vi "GetText.vi"(8 "error in":errorcluster, 11 "Thermo Channel in":refnum<class "Thermo Channel.lvclass">) -> (0 "error out":errorcluster, 1 "additional text":string, 2 "text":string, 3 "Thermo Channel out":refnum<class "Thermo Channel.lvclass">, 4 "glyph":string)   [LabVIEW 2025, in "Thermo.lvlib" / "Thermo Channel.lvclass"]
doc: "Copyright 2017 National Instruments Corporation\n\nLicensed under the Apache License, Version 2.0 (the \"License\"); you may not use this file except in compliance with the License. You may obtain a copy of the License at http://www.apache.org/licenses/LICENSE-2.0\nUnless required by applicable law or agreed to in writing, software distributed under the License is distributed on an \"AS IS\" BASIS, WITHOUT WARRANTIES OR CONDITIONS OF ANY KIND, either express or implied. See the License for the specific language governing permissions and limitations under the License."
uses:
  Thermo Channel.lvclass
  Thermo Channel.lvclass/Thermo Channel.ctl
  Thermo Channel configuration/Thermo Channel configuration.lvclass
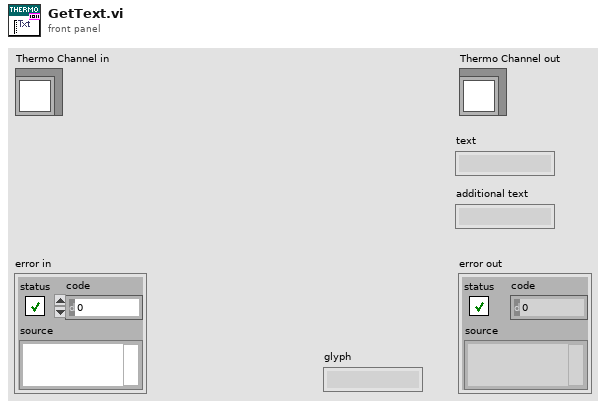
[diagram p1: front panel]
types:
  T1 = typedef "Abstract Engine.lvlibp/Channel configuration.lvclass/Default Channel.ctl" = cluster{"Address":string, "SW Alias":string, "Enabled":bool, "Type":string, "Description":string}
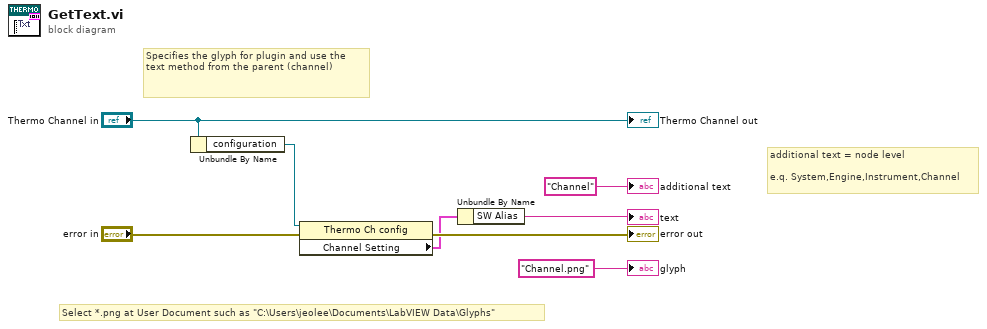
[diagram p0: block diagram]
diagram:
  # "Select *.png at User Document such as \"C:\\Users\\jeolee\\Documents\\LabVIEW Data\\Glyphs\""
  # "additional text = node level\n\ne.q. System,Engine,Instrument,Channel"
  # "Specifies the glyph for plugin and use the text method from the parent (channel)"
  n1 = Unbundle By Name("Thermo Channel in") -> ("configuration"=w4:refnum<class "Thermo Channel configuration.lvclass">)
  n2 = property class="Thermo Ch config"(reference=w4, error in="error in") -> (error out=→"error out":errorcluster, "Channel Setting"=w1:T1)  [unwired: 1 out]
  n3 = Unbundle By Name(w1) -> ("SW Alias"=→"text":string)
  "Thermo Channel out" <- "Thermo Channel in"
  "additional text" <- "Channel" ("additional text")
  "glyph" <- "Channel.png" ("glyph")
